vi "motor set angle.vi"(8 "error in (no error)":errorcluster, 11 "angle":dbl) -> (0 "error out":errorcluster)   [LabVIEW 2013]
uses:
  private/motor global state actions.ctl
panel:
  out "Initial error state":bool
  out "LabJack Error Message":string
  # "Rotates the sample rod to an (absolute) angle."
  # "0° = end switch activated.\nUse only positive values here!"
  # "If motor does not react after \nsuccessfull initialization \n&  RED lamp at power supply, \nswitch OFF powersupply,\nWAIT 30s and turn ON again."
  # "NEVER exceed 320° !!!\nEnsure that cables can follow \nstage movement !!!"
  # "(Power is probably off)"
  # "Error sources in general: \n- voltage < 40 V (Power Source OFF,\nNetzschwankung...)\n- Endstufe > 58°C\n- I too high (unprobable)\n(see ZSO 92_70 manual)"
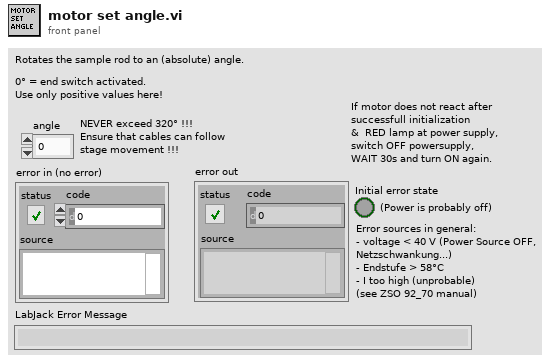
[diagram p1: front panel]
types:
  T1 = typedef "motor global state actions.ctl" = enum16{"set value", "get value", "set angle", "set initialized", "set complete", "set handle", "get handle"}
  T2 = typedef "motor global state control.ctl" = cluster{"current angle":dbl, "initialized":bool, "completed":bool, "Handle":i32}
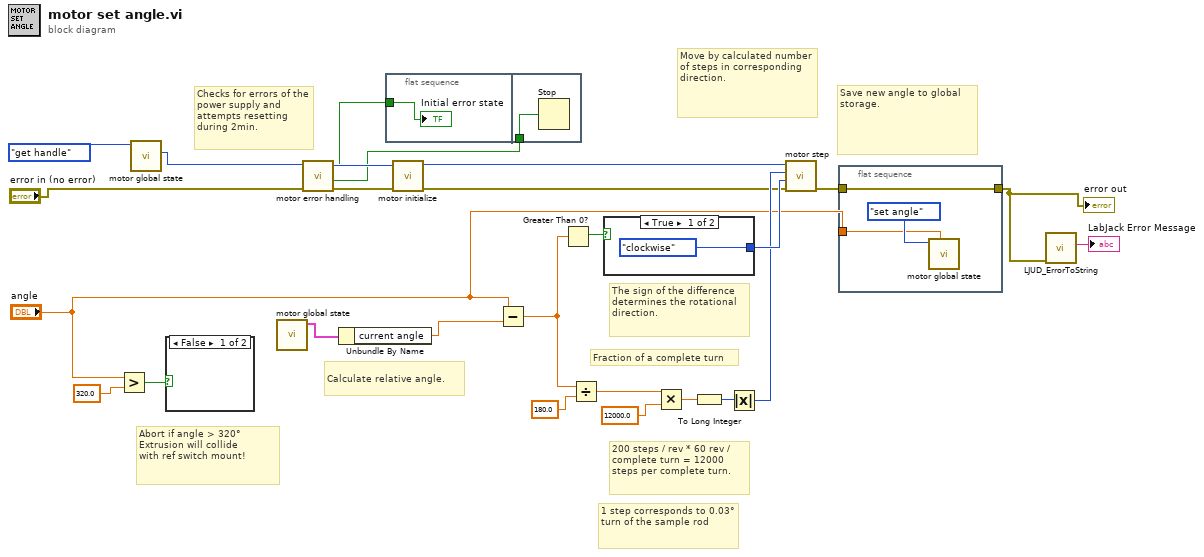
[diagram p0: block diagram]
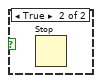
[diagram p2: hidden frame]
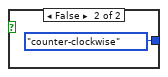
[diagram p3: hidden frame]
diagram:
  # "Checks for errors of the power supply and attempts resetting during 2min."
  # "1 step corresponds to 0.03° turn of the sample rod"
  # "Abort if angle > 320°\nExtrusion will collide \nwith ref switch mount!"
  # "Fraction of a complete turn"
  # "Save new angle to global storage."
  # "Move by calculated number of steps in corresponding direction."
  # "200 steps / rev * 60 rev / complete turn = 12000 steps per complete turn."
  # "The sign of the difference determines the rotational direction."
  # "Calculate relative angle."
  n1 = Greater?(x="angle", y=320.0) -> (0:w11:bool)
  n2 = call "motor global state.vi"("action"=motor_global_state_actions."get handle") -> ("Handle Out"=w7:i32)  [unwired: 9 in, 1 out]
  n3 = case shown="False" w11 {
    frame False {
    }
    frame True {
      n4 = Stop() -> ()  [unwired: 1 in]
    }
  }
  n5 = call "motor global state.vi"() -> ("motor global state"=w19:T2)  [unwired: 10 in, 1 out]
  n6 = call "motor error handling.vi"("error in (no error)"="error in (no error)", "Handle in"=w7) -> ("error out"=w4:errorcluster, "Stop .vi?"=w2:bool, "Handle Out out"=w5:i32, "Error state"=w3:bool)  [unwired: 6 in]
  n7 = Unbundle By Name(w19) -> ("current angle"=w1:dbl)
  n8 = flat-sequence {
    tunnel: w3 -> [w27]
    tunnel: w2 -> [w28]
    frame #0 {
      "Initial error state" <- w27
    }
    frame #1 {
      n9 = Stop(stop? (T)=w28) -> ()
    }
  }
  n10 = call "motor initialize.vi"("error in (no error)"=w4, "Handle In"=w5) -> ("error out"=w8:errorcluster, "Handle Out"=w9:i32)  [unwired: 8 in]
  n11 = Subtract(x="angle", y=w1) -> (x-y=w15:dbl)
  n12 = Greater Than 0?(x=w15) -> (x > 0?=w26:bool)
  n13 = Divide(x=w15, y=180.0) -> (x/y=w23:dbl)
  n14 = case shown="True" w26 {
    tunnel: [enum16{"counter-clockwise", "clockwise"}."clockwise" ("direction") enum16{"counter-clockwise", "clockwise"}."counter-clockwise" ("direction")] -> w17
    frame True {
    }
    frame False {
    }
  }
  n15 = Multiply(x=w23, y=12000.0) -> (x*y=w24:dbl)
  n16 = To Long Integer(number=w24) -> (32bit integer=w21:i32)
  n17 = Absolute Value(x=w21) -> (abs(x)=w16:i32)
  n18 = call "motor step.vi"("error in (no error)"=w8, "direction"=w17, "steps"=w16, "Handle In"=w9) -> ("error out"=w18:errorcluster)  [unwired: 4 in, 3 out]
  n19 = flat-sequence {
    tunnel: w18 -> [w33]
    tunnel: [w33] -> w10
    tunnel: "angle" -> [w31]
    frame #0 {
      n20 = call "motor global state.vi"("angle"=w31, "action"=motor_global_state_actions."set angle" ("Motor FGV actions")) -> ()  [unwired: 8 in, 2 out]
    }
  }
  n21 = call <vilib>:"LJUD_ErrorToString.vi"("error in"=w10) -> ("String"=→"LabJack Error Message":string)  [unwired: 10 in]
  "error out" <- w10
